vi "MoveRudderInEmergency.vi"(11 "ForceOnRudder":dbl) -> (3 "EmergencyRudderSetting":T1 min=-1.0 max=1.0)   [LabVIEW 2012]
doc: "Intended to move the rudder to reduce force on it in moments of extremely high stress, this should be done after the nature of the 'Force on the rudder' value is determined, not just it's magnitude but also it's behavior in turns and other characteristics.\n\nEric Schneider, Jan. 2014"
uses:
  Data/TypeDefs/Rudder Set Suggestions.ctl
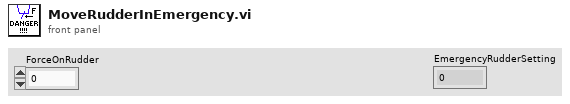
[diagram p1: front panel]
types:
  T1 = typedef "Rudder Set Suggestions.ctl" = dbl
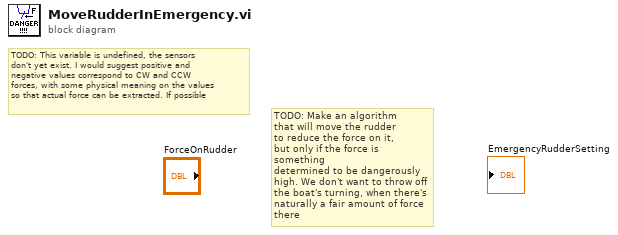
[diagram p0: block diagram]
diagram:
  # "TODO: Make an algorithm\nthat will move the rudder\nto reduce the force on it,\nbut only if the force is something\ndetermined to be dangerously\nhigh. We don't want to throw off\nthe boat's turning, when there's\nnaturally a fair amount of force\nthere"
  # "TODO: This variable is undefined, the sensors\ndon't yet exist. I would suggest positive and\nnegative values correspond to CW and CCW\nforces, with some physical meaning on the values\nso that actual force can be extracted. If possible"
